vi "Get Register.vi"(11 "jettl Actor in":refnum<class "jettl Actor.lvclass">) -> (2 "Register":refnum<event-registration>)   [LabVIEW 2021, in "jettl.lvlib" / "Temporary Actor.lvlib" / "jettl Actor.lvclass"]
uses:
  jettl Actor.lvclass
  Msg/Msg.lvclass
  jettl Actor.lvclass/jettl Actor.ctl
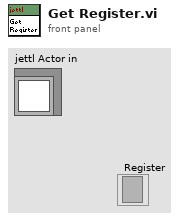
[diagram p1: front panel]
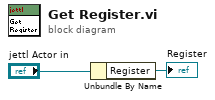
[diagram p0: block diagram]
diagram:
  n1 = Unbundle By Name("jettl Actor in") -> ("Register"=→"Register":refnum<event-registration>)
